vi "Main.vi"(7 "sweep rate, /min":dbl=0.2, 8 "sweep to:":dbl=-0.5, 9 "sweep":T6(radio)=enum."time_sweep") -> ()   [LabVIEW 2017] (continued)
                    n2924 = Build Array(w3784) -> (w3785:string[])
                    n2925 = property on="data_caption" class="Str"("Value"=w3787) -> ()  [unwired: 2 in, 2 out]
                    n2926 = property on="Figure_axis" class="Arr (strict)"("Value"=w3785) -> ()  [unwired: 2 in, 2 out]
                  }
                }
              }
              frame "2636a_smub" {
                n2927 = stacked-sequence {
                  frame #0 {
                    n2928 = property on="data_caption" class="Str"("Value"="") -> ()  [unwired: 2 in, 2 out]
                    n2929 = property on="Figure_axis" class="Arr (strict)"("Value"=string[] [] ("Figure_axis_string")) -> ()  [unwired: 2 in, 2 out]
                  }
                  frame #1 {
                    w3790 = "V_sweep_2636a_smub" ("V_sweep")
                    n2930 = Build Array(w3790) -> (w3791:string[])
                    n2931 = Concatenate Strings(w3790, "\t") -> (w3793:string)
                    n2932 = property on="Figure_axis" class="Arr (strict)"("Value"=w3791) -> ()  [unwired: 2 in, 2 out]
                    n2933 = property on="data_caption" class="Str"("Value"=w3793) -> ()  [unwired: 2 in, 2 out]
                  }
                }
              }
              frame "time_sweep", Default {
                n2934 = stacked-sequence {
                  frame #0 {
                    n2935 = property on="data_caption" class="Str"("Value"="") -> ()  [unwired: 2 in, 2 out]
                    n2936 = property on="Figure_axis" class="Arr (strict)"("Value"=string[] [] ("Figure_axis_string")) -> ()  [unwired: 2 in, 2 out]
                  }
                  frame #1 {
                    w3796 = "time_sweep" ("V_sweep")
                    n2937 = Build Array(w3796) -> (w3797:string[])
                    n2938 = Concatenate Strings(w3796, "\t") -> (w3798:string)
                    n2939 = property on="Figure_axis" class="Arr (strict)"("Value"=w3797) -> ()  [unwired: 2 in, 2 out]
                    n2940 = property on="data_caption" class="Str"("Value"=w3798) -> ()  [unwired: 2 in, 2 out]
                  }
                }
              }
              frame "iPS" {
                n2941 = stacked-sequence {
                  frame #0 {
                    n2942 = property on="data_caption" class="Str"("Value"="") -> ()  [unwired: 2 in, 2 out]
                    n2943 = property on="Figure_axis" class="Arr (strict)"("Value"=string[] [] ("Figure_axis_string")) -> ()  [unwired: 2 in, 2 out]
                  }
                  frame #1 {
                    w3802 = "Teslatron_iPS_OutputField" ("V_sweep")
                    n2944 = Build Array(w3802) -> (w3803:string[])
                    n2945 = Concatenate Strings(w3802, "\t") -> (w3805:string)
                    n2946 = property on="Figure_axis" class="Arr (strict)"("Value"=w3803) -> ()  [unwired: 2 in, 2 out]
                    n2947 = property on="data_caption" class="Str"("Value"=w3805) -> ()  [unwired: 2 in, 2 out]
                  }
                }
              }
              frame "iTC" {
                n2948 = stacked-sequence {
                  frame #0 {
                    n2949 = property on="data_caption" class="Str"("Value"="") -> ()  [unwired: 2 in, 2 out]
                    n2950 = property on="Figure_axis" class="Arr (strict)"("Value"=string[] ["", "SR830_1_ip", "SR830_1_oop", "SR830_2_ip", "SR830_2_oop", "2461_meas_v", "2461_meas_i", "2636A_smua_v", "2636A_smua_i", "formula"] ("Figure_axis")) -> ()  [unwired: 2 in, 2 out]
                  }
                  frame #1 {
                    w3810 = "Teslatron_iTC_Temp"
                    n2951 = Build Array(w3810) -> (w3809:string[])
                    n2952 = Concatenate Strings(w3810, "\t") -> (w3808:string)
                    n2953 = property on="data_caption" class="Str"("Value"=w3808) -> ()  [unwired: 2 in, 2 out]
                    n2954 = property on="Figure_axis" class="Arr (strict)"("Value"=w3809) -> ()  [unwired: 2 in, 2 out]
                  }
                }
              }
              frame "2461" {
                n2955 = stacked-sequence {
                  frame #0 {
                    n2956 = property on="data_caption" class="Str"("Value"="") -> ()  [unwired: 2 in, 2 out]
                    n2957 = property on="Figure_axis" class="Arr (strict)"("Value"=string[] ["", "SR830_1_ip", "SR830_1_oop", "SR830_2_ip", "SR830_2_oop", "2461_meas_v", "2461_meas_i", "2636A_smua_v", "2636A_smua_i", "formula"] ("Figure_axis")) -> ()  [unwired: 2 in, 2 out]
                  }
                  frame #1 {
                    w3816 = "I_sweep_2461"
                    n2958 = Build Array(w3816) -> (w3815:string[])
                    n2959 = Concatenate Strings(w3816, "\t") -> (w3814:string)
                    n2960 = property on="data_caption" class="Str"("Value"=w3814) -> ()  [unwired: 2 in, 2 out]
                    n2961 = property on="Figure_axis" class="Arr (strict)"("Value"=w3815) -> ()  [unwired: 2 in, 2 out]
                  }
                }
              }
            }
            n2962 = case shown="True" w3759 {
              frame False {
              }
              frame True {
                # "opens session for 2636a system sourcemeter"
                n2963 = local read "2336A addr"() -> (w3818:refnum<visa-resource-name>)
                n2964 = VISA Open(VISA resource name=w3818) -> ()  [unwired: 4 in, 2 out]
              }
            }
          }
          frame #1 {
            # "this part constructs the first (text) line for the data file with names of all measured variables,\nalso constructs a text array contaning names of all measured variable for the \"ring\" (so parameter can be selected and plotted)"
            n2965 = stacked-sequence {
              tunnel: [w3819 _ _ _ _ _ _ _ _ _ _ _ _ _ _ _ _ _ _ _ _ _ _ _ _ _ _ _ _ _ _ _ _ _ _ _ _ _ _ _ _ _ _ _ _ _ _ _ _ _ _ _] -> _
              frame #0 {
                # "SR830 1 in phase (SR830_1_ip)"
                n2966 = local read "SR830 1 ip"() -> (w3824:bool)
                n2967 = property on="Figure_axis" class="Arr (strict)"() -> ("Value"=w3821:string[])  [unwired: 2 in, 2 out]
                n2968 = property on="data_caption" class="Str"() -> ("Value"=w3823:string)  [unwired: 2 in, 2 out]
                n2969 = case shown="True" w3824 {
                  tunnel: w3823 -> [w3826 w3832]
                  tunnel: [w3826 w3831] -> w3822
                  tunnel: w3821 -> [w3825 w3829]
                  tunnel: [w3825 w3827] -> w3820
                  frame False {
                    # "not measure SR830 1 in phase signal (SR830_1_ip)"
                  }
                  frame True {
                    w3828 = "SR830_1_ip"
                    # "measure SR830 1 in phase signal (SR830_1_ip)"
                    n2970 = local read "SR830 1 addr"() -> (w3833:u8)
                    n2971 = Number To Decimal String(number=w3833) -> (decimal integer string=w3834:string)  [unwired: 1 in]
                    n2972 = GPIB Clear(3:w3834) -> ()  [unwired: 1 in, 2 out]
                    n2973 = Build Array (concatenate)(w3829, w3828) -> (w3827:string[])
                    n2974 = Concatenate Strings(w3832, w3828, "\t") -> (w3831:string)
                  }
                }
                n2975 = property on="Figure_axis" class="Arr (strict)"("Value"=w3820) -> ()  [unwired: 2 in, 2 out]
                n2976 = property on="data_caption" class="Str"("Value"=w3822) -> (error out=w3819:errorcluster)  [unwired: 2 in, 1 out]
              }
              frame #1 {
                # "SR830 1 out of phase (SR830_1_oop)"
                n2977 = local read "SR830 1 oop"() -> (w3839:bool)
                n2978 = property on="Figure_axis" class="Arr (strict)"() -> ("Value"=w3836:string[])  [unwired: 2 in, 2 out]
                n2979 = property on="data_caption" class="Str"() -> ("Value"=w3838:string)  [unwired: 2 in, 2 out]
                n2980 = case shown="False" w3839 {
                  tunnel: w3838 -> [w3841 w3847]
                  tunnel: [w3841 w3846] -> w3837
                  tunnel: w3836 -> [w3840 w3844]
                  tunnel: [w3840 w3842] -> w3835
                  frame False {
                    # "not measure SR830 1 out of phase signal (SR830_1_oop)"
                  }
                  frame True {
                    w3843 = "SR830_1_oop"
                    # "measure SR830 1 out of phase signal (SR830_1_oop)"
                    n2981 = local read "SR830 1 addr"() -> (w3848:u8)
                    n2982 = Number To Decimal String(number=w3848) -> (decimal integer string=w3849:string)  [unwired: 1 in]
                    n2983 = GPIB Clear(3:w3849) -> ()  [unwired: 1 in, 2 out]
                    n2984 = Build Array (concatenate)(w3844, w3843) -> (w3842:string[])
                    n2985 = Concatenate Strings(w3847, w3843, "\t") -> (w3846:string)
                  }
                }
                n2986 = property on="Figure_axis" class="Arr (strict)"("Value"=w3835) -> ()  [unwired: 2 in, 2 out]
                n2987 = property on="data_caption" class="Str"("Value"=w3837) -> ()  [unwired: 2 in, 2 out]
              }
              frame #2 {
                # "SR830 2 in phase (SR830_2_ip)"
                n2988 = local read "SR830 2 ip"() -> (w3854:bool)
                n2989 = property on="Figure_axis" class="Arr (strict)"() -> ("Value"=w3851:string[])  [unwired: 2 in, 2 out]
                n2990 = property on="data_caption" class="Str"() -> ("Value"=w3853:string)  [unwired: 2 in, 2 out]
                n2991 = case shown="True" w3854 {
                  tunnel: w3853 -> [w3856 w3862]
                  tunnel: [w3856 w3861] -> w3852
                  tunnel: w3851 -> [w3855 w3859]
                  tunnel: [w3855 w3857] -> w3850
                  frame False {
                    # "not measure SR830 2 in phase signal (SR830_2_ip)"
                  }
                  frame True {
                    w3858 = "SR830_2_ip"
                    # "measure SR830 2 in phase signal (SR830_2_ip)"
                    n2992 = local read "SR830 2 addr"() -> (w3863:u8)
                    n2993 = Number To Decimal String(number=w3863) -> (decimal integer string=w3864:string)  [unwired: 1 in]
                    n2994 = GPIB Clear(3:w3864) -> ()  [unwired: 1 in, 2 out]
                    n2995 = Build Array (concatenate)(w3859, w3858) -> (w3857:string[])
                    n2996 = Concatenate Strings(w3862, w3858, "\t") -> (w3861:string)
                  }
                }
                n2997 = property on="Figure_axis" class="Arr (strict)"("Value"=w3850) -> ()  [unwired: 2 in, 2 out]
                n2998 = property on="data_caption" class="Str"("Value"=w3852) -> ()  [unwired: 2 in, 2 out]
              }
              frame #3 {
                # "SR830 2 out of phase (SR830_2_oop)"
                n2999 = local read "SR830 2 oop"() -> (w3869:bool)
                n3000 = property on="Figure_axis" class="Arr (strict)"() -> ("Value"=w3866:string[])  [unwired: 2 in, 2 out]
                n3001 = property on="data_caption" class="Str"() -> ("Value"=w3868:string)  [unwired: 2 in, 2 out]
                n3002 = case shown="False" w3869 {
                  tunnel: w3868 -> [w3871 w3877]
                  tunnel: [w3871 w3876] -> w3867
                  tunnel: w3866 -> [w3870 w3874]
                  tunnel: [w3870 w3872] -> w3865
                  frame False {
                    # "not measure SR830 2 out of phase signal (SR830_2_oop)"
                  }
                  frame True {
                    w3873 = "SR830_2_oop"
                    # "measure SR830 2 out of phase signal (SR830_2_oop)"
                    n3003 = local read "SR830 2 addr"() -> (w3878:u8)
                    n3004 = Number To Decimal String(number=w3878) -> (decimal integer string=w3879:string)  [unwired: 1 in]
                    n3005 = GPIB Clear(3:w3879) -> ()  [unwired: 1 in, 2 out]
                    n3006 = Build Array (concatenate)(w3874, w3873) -> (w3872:string[])
                    n3007 = Concatenate Strings(w3877, w3873, "\t") -> (w3876:string)
                  }
                }
                n3008 = property on="Figure_axis" class="Arr (strict)"("Value"=w3865) -> ()  [unwired: 2 in, 2 out]
                n3009 = property on="data_caption" class="Str"("Value"=w3867) -> ()  [unwired: 2 in, 2 out]
              }
              frame #4 {
                # "SR830 3 in phase (SR830_3_ip)"
                n3010 = local read "SR830 3 ip"() -> (w3884:bool)
                n3011 = property on="Figure_axis" class="Arr (strict)"() -> ("Value"=w3881:string[])  [unwired: 2 in, 2 out]
                n3012 = property on="data_caption" class="Str"() -> ("Value"=w3883:string)  [unwired: 2 in, 2 out]
                n3013 = case shown="True" w3884 {
                  tunnel: w3883 -> [w3886 w3892]
                  tunnel: [w3886 w3891] -> w3882
                  tunnel: w3881 -> [w3885 w3889]
                  tunnel: [w3885 w3887] -> w3880
                  frame False {
                    # "not measure SR830 3 in phase signal (SR830_3_ip)"
                  }
                  frame True {
                    w3888 = "SR830_3_ip"
                    # "measure SR830 3 in phase signal (SR830_3_ip)"
                    n3014 = local read "SR830 3 addr"() -> (w3893:u8)
                    n3015 = Number To Decimal String(number=w3893) -> (decimal integer string=w3894:string)  [unwired: 1 in]
                    n3016 = GPIB Clear(3:w3894) -> ()  [unwired: 1 in, 2 out]
                    n3017 = Build Array (concatenate)(w3889, w3888) -> (w3887:string[])
                    n3018 = Concatenate Strings(w3892, w3888, "\t") -> (w3891:string)
                  }
                }
                n3019 = property on="Figure_axis" class="Arr (strict)"("Value"=w3880) -> ()  [unwired: 2 in, 2 out]
                n3020 = property on="data_caption" class="Str"("Value"=w3882) -> ()  [unwired: 2 in, 2 out]
              }
              frame #5 {
                # "SR830 3 out of phase (SR830_3_oop)"
                n3021 = local read "SR830 3 oop"() -> (w3899:bool)
                n3022 = property on="Figure_axis" class="Arr (strict)"() -> ("Value"=w3896:string[])  [unwired: 2 in, 2 out]
                n3023 = property on="data_caption" class="Str"() -> ("Value"=w3898:string)  [unwired: 2 in, 2 out]
                n3024 = case shown="True" w3899 {
                  tunnel: w3898 -> [w3901 w3907]
                  tunnel: [w3901 w3906] -> w3897
                  tunnel: w3896 -> [w3900 w3904]
                  tunnel: [w3900 w3902] -> w3895
                  frame False {
                    # "not measure SR830 3 out of phase signal (SR830_3_oop)"
                  }
                  frame True {
                    w3903 = "SR830_3_oop"
                    # "measure SR830 3 out phase signal (SR830_3_oop)"
                    n3025 = local read "SR830 3 addr"() -> (w3908:u8)
                    n3026 = Number To Decimal String(number=w3908) -> (decimal integer string=w3909:string)  [unwired: 1 in]
                    n3027 = GPIB Clear(3:w3909) -> ()  [unwired: 1 in, 2 out]
                    n3028 = Build Array (concatenate)(w3904, w3903) -> (w3902:string[])
                    n3029 = Concatenate Strings(w3907, w3903, "\t") -> (w3906:string)
                  }
                }
                n3030 = property on="Figure_axis" class="Arr (strict)"("Value"=w3895) -> ()  [unwired: 2 in, 2 out]
                n3031 = property on="data_caption" class="Str"("Value"=w3897) -> ()  [unwired: 2 in, 2 out]
              }
              frame #6 {
                # "SR830 4 in phase (SR830_4_ip)"
                n3032 = local read "SR830 4 ip"() -> (w3914:bool)
                n3033 = property on="Figure_axis" class="Arr (strict)"() -> ("Value"=w3911:string[])  [unwired: 2 in, 2 out]
                n3034 = property on="data_caption" class="Str"() -> ("Value"=w3913:string)  [unwired: 2 in, 2 out]
                n3035 = case shown="False" w3914 {
                  tunnel: w3913 -> [w3916 w3922]
                  tunnel: [w3916 w3921] -> w3912
                  tunnel: w3911 -> [w3915 w3919]
                  tunnel: [w3915 w3917] -> w3910
                  frame False {
                    # "not measure SR830 4 in phase signal (SR830_4_ip)"
                  }
                  frame True {
                    w3918 = "SR830_4_ip"
                    # "measure SR830 4 in phase signal (SR830_4_ip)"
                    n3036 = local read "SR830 4 addr"() -> (w3923:u8)
                    n3037 = Number To Decimal String(number=w3923) -> (decimal integer string=w3924:string)  [unwired: 1 in]
                    n3038 = GPIB Clear(3:w3924) -> ()  [unwired: 1 in, 2 out]
                    n3039 = Build Array (concatenate)(w3919, w3918) -> (w3917:string[])
                    n3040 = Concatenate Strings(w3922, w3918, "\t") -> (w3921:string)
                  }
                }
                n3041 = property on="Figure_axis" class="Arr (strict)"("Value"=w3910) -> ()  [unwired: 2 in, 2 out]
                n3042 = property on="data_caption" class="Str"("Value"=w3912) -> ()  [unwired: 2 in, 2 out]
              }
              frame #7 {
                # "SR830 4 out of phase (SR830_4_oop)"
                n3043 = local read "SR830 4 oop"() -> (w3929:bool)
                n3044 = property on="Figure_axis" class="Arr (strict)"() -> ("Value"=w3926:string[])  [unwired: 2 in, 2 out]
                n3045 = property on="data_caption" class="Str"() -> ("Value"=w3928:string)  [unwired: 2 in, 2 out]
                n3046 = case shown="False" w3929 {
                  tunnel: w3928 -> [w3931 w3937]
                  tunnel: [w3931 w3936] -> w3927
                  tunnel: w3926 -> [w3930 w3934]
                  tunnel: [w3930 w3932] -> w3925
                  frame False {
                    # "not measure SR830 4 out of phase signal (SR830_4_oop)"
                  }
                  frame True {
                    w3933 = "SR830_4_oop"
                    # "measure SR830 4 out of phase signal (SR830_4_oop)"
                    n3047 = local read "SR830 4 addr"() -> (w3938:u8)
                    n3048 = Number To Decimal String(number=w3938) -> (decimal integer string=w3939:string)  [unwired: 1 in]
                    n3049 = GPIB Clear(3:w3939) -> ()  [unwired: 1 in, 2 out]
                    n3050 = Build Array (concatenate)(w3934, w3933) -> (w3932:string[])
                    n3051 = Concatenate Strings(w3937, w3933, "\t") -> (w3936:string)
                  }
                }
                n3052 = property on="Figure_axis" class="Arr (strict)"("Value"=w3925) -> ()  [unwired: 2 in, 2 out]
                n3053 = property on="data_caption" class="Str"("Value"=w3927) -> ()  [unwired: 2 in, 2 out]
              }
              frame #8 {
                # "SR830 5 in phase (SR830_5_ip)"
                n3054 = local read "SR830 5 ip"() -> (w3944:bool)
                n3055 = property on="Figure_axis" class="Arr (strict)"() -> ("Value"=w3941:string[])  [unwired: 2 in, 2 out]
                n3056 = property on="data_caption" class="Str"() -> ("Value"=w3943:string)  [unwired: 2 in, 2 out]
                n3057 = case shown="True" w3944 {
                  tunnel: w3943 -> [w3946 w3952]
                  tunnel: [w3946 w3951] -> w3942
                  tunnel: w3941 -> [w3945 w3949]
                  tunnel: [w3945 w3947] -> w3940
                  frame False {
                    # "not measure SR830 5 in phase signal (SR830_5_ip)"
                  }
                  frame True {
                    w3948 = "SR830_5_ip"
                    # "measure SR830 5 in phase signal (SR830_5_ip)"
                    n3058 = local read "SR830 5 addr"() -> (w3953:u8)
                    n3059 = Number To Decimal String(number=w3953) -> (decimal integer string=w3954:string)  [unwired: 1 in]
                    n3060 = GPIB Clear(3:w3954) -> ()  [unwired: 1 in, 2 out]
                    n3061 = Build Array (concatenate)(w3949, w3948) -> (w3947:string[])
                    n3062 = Concatenate Strings(w3952, w3948, "\t") -> (w3951:string)
                  }
                }
                n3063 = property on="Figure_axis" class="Arr (strict)"("Value"=w3940) -> ()  [unwired: 2 in, 2 out]
                n3064 = property on="data_caption" class="Str"("Value"=w3942) -> ()  [unwired: 2 in, 2 out]
              }
              frame #9 {
                # "SR830 5 out of phase (SR830_5_oop)"
                n3065 = local read "SR830 5 oop"() -> (w3959:bool)
                n3066 = property on="Figure_axis" class="Arr (strict)"() -> ("Value"=w3956:string[])  [unwired: 2 in, 2 out]
                n3067 = property on="data_caption" class="Str"() -> ("Value"=w3958:string)  [unwired: 2 in, 2 out]
                n3068 = case shown="True" w3959 {
                  tunnel: w3958 -> [w3961 w3967]
                  tunnel: [w3961 w3966] -> w3957
                  tunnel: w3956 -> [w3960 w3964]
                  tunnel: [w3960 w3962] -> w3955
                  frame False {
                    # "not measure SR830 5 out of phase signal (SR830_5_oop)"
                  }
                  frame True {
                    w3963 = "SR830_5_oop"
                    # "measure SR830 5 out of phase signal (SR830_5_oop)"
                    n3069 = local read "SR830 5 addr"() -> (w3968:u8)
                    n3070 = Number To Decimal String(number=w3968) -> (decimal integer string=w3969:string)  [unwired: 1 in]
                    n3071 = GPIB Clear(3:w3969) -> ()  [unwired: 1 in, 2 out]
                    n3072 = Build Array (concatenate)(w3964, w3963) -> (w3962:string[])
                    n3073 = Concatenate Strings(w3967, w3963, "\t") -> (w3966:string)
                  }
                }
                n3074 = property on="Figure_axis" class="Arr (strict)"("Value"=w3955) -> ()  [unwired: 2 in, 2 out]
                n3075 = property on="data_caption" class="Str"("Value"=w3957) -> ()  [unwired: 2 in, 2 out]
              }
              frame #10 {
                # "SR830 6 in phase (SR830_6_ip)"
                n3076 = property on="SR830_6_ip" class="Bool (strict)"() -> ("Value"=w3970:bool)  [unwired: 2 in, 2 out]
                n3077 = property on="Figure_axis" class="Arr (strict)"() -> ("Value"=w3972:string[])  [unwired: 2 in, 2 out]
                n3078 = property on="data_caption" class="Str"() -> ("Value"=w3974:string)  [unwired: 2 in, 2 out]
                n3079 = case shown="True" w3970 {
                  tunnel: w3974 -> [w3976 w3982]
                  tunnel: [w3976 w3981] -> w3973
                  tunnel: w3972 -> [w3975 w3979]
                  tunnel: [w3975 w3977] -> w3971
                  frame False {
                    # "not measure SR830 6 in phase signal (SR830_6_ip)"
                  }
                  frame True {
                    w3978 = "SR830_6_ip"
                    # "measure SR830 6 in phase signal (SR830_6_ip)"
                    n3080 = local read "SR830_6"() -> (w3983:u8)
                    n3081 = Number To Decimal String(number=w3983) -> (decimal integer string=w3984:string)  [unwired: 1 in]
                    n3082 = GPIB Clear(3:w3984) -> ()  [unwired: 1 in, 2 out]
                    n3083 = Build Array (concatenate)(w3979, w3978) -> (w3977:string[])
                    n3084 = Concatenate Strings(w3982, w3978, "\t") -> (w3981:string)
                  }
                }
                n3085 = property on="Figure_axis" class="Arr (strict)"("Value"=w3971) -> ()  [unwired: 2 in, 2 out]
                n3086 = property on="data_caption" class="Str"("Value"=w3973) -> ()  [unwired: 2 in, 2 out]
              }
              frame #11 {
                # "SR830 6 out of phase (SR830_6_oop)"
                n3087 = local read "SR830_6_oop"() -> (w3989:bool)
                n3088 = property on="Figure_axis" class="Arr (strict)"() -> ("Value"=w3986:string[])  [unwired: 2 in, 2 out]
                n3089 = property on="data_caption" class="Str"() -> ("Value"=w3988:string)  [unwired: 2 in, 2 out]
                n3090 = case shown="False" w3989 {
                  tunnel: w3988 -> [w3991 w3997]
                  tunnel: [w3991 w3996] -> w3987
                  tunnel: w3986 -> [w3990 w3994]
                  tunnel: [w3990 w3992] -> w3985
                  frame False {
                    # "not measure SR830 6 out of phase signal (SR830_6_oop)"
                  }
                  frame True {
                    w3993 = "SR830_6_oop"
                    # "measure SR830 6 out of phase signal (SR830_6_oop)"
                    n3091 = local read "SR830_6"() -> (w3998:u8)
                    n3092 = Number To Decimal String(number=w3998) -> (decimal integer string=w3999:string)  [unwired: 1 in]
                    n3093 = GPIB Clear(3:w3999) -> ()  [unwired: 1 in, 2 out]
                    n3094 = Build Array (concatenate)(w3994, w3993) -> (w3992:string[])
                    n3095 = Concatenate Strings(w3997, w3993, "\t") -> (w3996:string)
                  }
                }
                n3096 = property on="Figure_axis" class="Arr (strict)"("Value"=w3985) -> ()  [unwired: 2 in, 2 out]
                n3097 = property on="data_caption" class="Str"("Value"=w3987) -> ()  [unwired: 2 in, 2 out]
              }
              frame #12 {
                # "SR830 7 in phase (SR830_7_ip)"
                n3098 = local read "SR830_7_ip"() -> (w4000:bool)
                n3099 = property on="Figure_axis" class="Arr (strict)"() -> ("Value"=w4002:string[])  [unwired: 2 in, 2 out]
                n3100 = property on="data_caption" class="Str"() -> ("Value"=w4004:string)  [unwired: 2 in, 2 out]
                n3101 = case shown="True" w4000 {
                  tunnel: w4004 -> [w4006 w4012]
                  tunnel: [w4006 w4011] -> w4003
                  tunnel: w4002 -> [w4005 w4009]
                  tunnel: [w4005 w4007] -> w4001
                  frame False {
                    # "not measure SR830 7 in phase signal (SR830_7_ip)"
                  }
                  frame True {
                    w4008 = "SR830_7_ip"
                    # "measure SR830 7 in phase signal (SR830_7_ip)"
                    n3102 = local read "SR830_7"() -> (w4013:u8)
                    n3103 = Number To Decimal String(number=w4013) -> (decimal integer string=w4014:string)  [unwired: 1 in]
                    n3104 = GPIB Clear(3:w4014) -> ()  [unwired: 1 in, 2 out]
                    n3105 = Build Array (concatenate)(w4009, w4008) -> (w4007:string[])
                    n3106 = Concatenate Strings(w4012, w4008, "\t") -> (w4011:string)
                  }
                }
                n3107 = property on="Figure_axis" class="Arr (strict)"("Value"=w4001) -> ()  [unwired: 2 in, 2 out]
                n3108 = property on="data_caption" class="Str"("Value"=w4003) -> ()  [unwired: 2 in, 2 out]
              }
              frame #13 {
                # "SR830 7 out of phase (SR830_7_oop)"
                n3109 = local read "SR830_7_oop"() -> (w4019:bool)
                n3110 = property on="Figure_axis" class="Arr (strict)"() -> ("Value"=w4016:string[])  [unwired: 2 in, 2 out]
                n3111 = property on="data_caption" class="Str"() -> ("Value"=w4018:string)  [unwired: 2 in, 2 out]
                n3112 = case shown="True" w4019 {
                  tunnel: w4018 -> [w4021 w4027]
                  tunnel: [w4021 w4026] -> w4017
                  tunnel: w4016 -> [w4020 w4024]
                  tunnel: [w4020 w4022] -> w4015
                  frame False {
                    # "not measure SR830 7 out of phase signal (SR830_7_oop)"
                  }
                  frame True {
                    w4023 = "SR830_7_oop"
                    # "measure SR830 7 out of phase signal (SR830_7_oop)"
                    n3113 = local read "SR830_7"() -> (w4028:u8)
                    n3114 = Number To Decimal String(number=w4028) -> (decimal integer string=w4029:string)  [unwired: 1 in]
                    n3115 = GPIB Clear(3:w4029) -> ()  [unwired: 1 in, 2 out]
                    n3116 = Build Array (concatenate)(w4024, w4023) -> (w4022:string[])
                    n3117 = Concatenate Strings(w4027, w4023, "\t") -> (w4026:string)
                  }
                }
                n3118 = property on="Figure_axis" class="Arr (strict)"("Value"=w4015) -> ()  [unwired: 2 in, 2 out]
                n3119 = property on="data_caption" class="Str"("Value"=w4017) -> ()  [unwired: 2 in, 2 out]
              }
              frame #14 {
                # "SR830 8 in phase (SR830_8_ip)"
                n3120 = local read "SR830_8_ip"() -> (w4030:bool)
                n3121 = property on="Figure_axis" class="Arr (strict)"() -> ("Value"=w4032:string[])  [unwired: 2 in, 2 out]
                n3122 = property on="data_caption" class="Str"() -> ("Value"=w4034:string)  [unwired: 2 in, 2 out]
                n3123 = case shown="True" w4030 {
                  tunnel: w4034 -> [w4036 w4042]
                  tunnel: [w4036 w4041] -> w4033
                  tunnel: w4032 -> [w4035 w4039]
                  tunnel: [w4035 w4037] -> w4031
                  frame False {
                    # "not measure SR830 8 in phase signal (SR830_8_ip)"
                  }
                  frame True {
                    w4038 = "SR830_8_ip"
                    # "measure SR830 8 in phase signal (SR830_8_ip)"
                    n3124 = local read "SR830_8"() -> (w4043:u8)
                    n3125 = Number To Decimal String(number=w4043) -> (decimal integer string=w4044:string)  [unwired: 1 in]
                    n3126 = GPIB Clear(3:w4044) -> ()  [unwired: 1 in, 2 out]
                    n3127 = Build Array (concatenate)(w4039, w4038) -> (w4037:string[])
                    n3128 = Concatenate Strings(w4042, w4038, "\t") -> (w4041:string)
                  }
                }
                n3129 = property on="Figure_axis" class="Arr (strict)"("Value"=w4031) -> ()  [unwired: 2 in, 2 out]
                n3130 = property on="data_caption" class="Str"("Value"=w4033) -> ()  [unwired: 2 in, 2 out]
              }
              frame #15 {
                # "SR830 8 out phase (SR830_8_oop)"
                n3131 = local read "SR830_8_oop"() -> (w4045:bool)
                n3132 = property on="Figure_axis" class="Arr (strict)"() -> ("Value"=w4047:string[])  [unwired: 2 in, 2 out]
                n3133 = property on="data_caption" class="Str"() -> ("Value"=w4049:string)  [unwired: 2 in, 2 out]
                n3134 = case shown="True" w4045 {
                  tunnel: w4049 -> [w4051 w4057]
                  tunnel: [w4051 w4056] -> w4048
                  tunnel: w4047 -> [w4050 w4054]
                  tunnel: [w4050 w4052] -> w4046
                  frame False {
                    # "not measure SR830 8 out phase signal (SR830_8_oop)"
                  }
                  frame True {
                    w4053 = "SR830_8_oop"
                    # "measure SR830 8 out phase signal (SR830_8_00p)"
                    n3135 = local read "SR830_8"() -> (w4058:u8)
                    n3136 = Number To Decimal String(number=w4058) -> (decimal integer string=w4059:string)  [unwired: 1 in]
                    n3137 = GPIB Clear(3:w4059) -> ()  [unwired: 1 in, 2 out]
                    n3138 = Build Array (concatenate)(w4054, w4053) -> (w4052:string[])
                    n3139 = Concatenate Strings(w4057, w4053, "\t") -> (w4056:string)
                  }
                }
                n3140 = property on="Figure_axis" class="Arr (strict)"("Value"=w4046) -> ()  [unwired: 2 in, 2 out]
                n3141 = property on="data_caption" class="Str"("Value"=w4048) -> ()  [unwired: 2 in, 2 out]
              }
              frame #16 {
                # "MFLI_V1"
                n3142 = property on="MFLI_1" class="Str" props=["Value"]() -> ()  [unwired: 2 in, 3 out]
                n3143 = property on="MFLI_V1" class="Bool (strict)"() -> ("Value"=w4060:bool)  [unwired: 2 in, 2 out]
                n3144 = property on="data_caption" class="Str"() -> ("Value"=w4064:string)  [unwired: 2 in, 2 out]
                n3145 = property on="Figure_axis" class="Arr (strict)"() -> ("Value"=w4062:string[])  [unwired: 2 in, 2 out]
                n3146 = case shown="True" w4060 {
                  tunnel: w4064 -> [w4066 w4076]
                  tunnel: [w4066 w4075] -> w4063
                  tunnel: w4062 -> [w4065 w4074]
                  tunnel: [w4065 w4073] -> w4061
                  frame False {
                    # "not measure 2461 voltage (2461_meas_v)"
                  }
                  frame True {
                    w4071 = "MFLI_Vy_1"
                    w4072 = "MFLI_Vx_1"
                    w4070 = "\t"
                    w4069 = "MFLI_freq_1"
                    n3147 = property on="HandleOut" class="Clust (strict)"() -> ("Value"=w4068:T5)  [unwired: 2 in, 2 out]
                    n3148 = Unbundle(w4068) -> ("Connected"=w4067:bool)  [unwired: 5 out]
                    n3149 = case shown="False" w4067 {
                      frame False {
                        n3150 = property on="MFLI_1" class="Str"() -> ("Value"=w4079:string)  [unwired: 2 in, 2 out]
                        n3151 = call <instrlib>:"ziOpen.vi"("Address"=w4079) -> ("HandleOut"=w4078:T5)  [unwired: 3 in, 2 out]
                        n3152 = call <instrlib>:"ziCheckVersion.vi"("Handle In"=w4078) -> ("Handle Out"=w4077:T5)  [unwired: 12 in, 2 out]
                        n3153 = property on="HandleOut" class="Clust (strict)"("Value"=w4077) -> ()  [unwired: 2 in, 2 out]
                      }
                      frame True {
                      }
                    }
                    n3154 = Build Array (concatenate)(w4074, w4072, w4071, w4069) -> (w4073:string[])
                    n3155 = Concatenate Strings(w4076, w4072, w4070, w4071, w4070, w4069, w4070) -> (w4075:string)
                  }
                }
                n3156 = property on="Figure_axis" class="Arr (strict)"("Value"=w4061) -> ()  [unwired: 2 in, 2 out]
                n3157 = property on="data_caption" class="Str"("Value"=w4063) -> ()  [unwired: 2 in, 2 out]
              }
              frame #17 {
                # "MFLI_I1"
                n3158 = property on="MFLI_I1" class="Bool (strict)"() -> ("Value"=w4080:bool)  [unwired: 2 in, 2 out]
                n3159 = property on="data_caption" class="Str"() -> ("Value"=w4084:string)  [unwired: 2 in, 2 out]
                n3160 = property on="Figure_axis" class="Arr (strict)"() -> ("Value"=w4082:string[])  [unwired: 2 in, 2 out]
                n3161 = case shown="True" w4080 {
                  tunnel: w4084 -> [w4086 w4096]
                  tunnel: [w4086 w4095] -> w4083
                  tunnel: w4082 -> [w4085 w4094]
                  tunnel: [w4085 w4093] -> w4081
                  frame False {
                    # "not measure 2461 voltage (2461_meas_v)"
                  }
                  frame True {
                    w4091 = "MFLI_Iy-1"
                    w4092 = "MFLI_Ix_1"
                    w4090 = "\t"
                    w4089 = "MFLI_freq_1"
                    n3162 = property on="HandleOut" class="Clust (strict)"() -> ("Value"=w4088:T5)  [unwired: 2 in, 2 out]
                    n3163 = Unbundle(w4088) -> ("Connected"=w4087:bool)  [unwired: 5 out]
                    n3164 = case shown="False" w4087 {
                      frame False {
                        n3165 = property on="MFLI_1" class="Str"() -> ("Value"=w4099:string)  [unwired: 2 in, 2 out]
                        n3166 = call <instrlib>:"ziOpen.vi"("Address"=w4099) -> ("HandleOut"=w4098:T5)  [unwired: 3 in, 2 out]
                        n3167 = call <instrlib>:"ziCheckVersion.vi"("Handle In"=w4098) -> ("Handle Out"=w4097:T5)  [unwired: 12 in, 2 out]
                        n3168 = property on="HandleOut" class="Clust (strict)"("Value"=w4097) -> ()  [unwired: 2 in, 2 out]
                      }
                      frame True {
                      }
                    }
                    n3169 = Build Array (concatenate)(w4094, w4092, w4091, w4089) -> (w4093:string[])
                    n3170 = Concatenate Strings(w4096, w4092, w4090, w4091, w4090, w4089, w4090) -> (w4095:string)
                  }
                }
                n3171 = property on="Figure_axis" class="Arr (strict)"("Value"=w4081) -> ()  [unwired: 2 in, 2 out]
                n3172 = property on="data_caption" class="Str"("Value"=w4083) -> ()  [unwired: 2 in, 2 out]
              }
              frame #18 {
                # "MFLI_V 2"
                n3173 = local read "MFLI_V2"() -> (w4100:bool)
                n3174 = property on="data_caption" class="Str"() -> ("Value"=w4104:string)  [unwired: 2 in, 2 out]
                n3175 = property on="Figure_axis" class="Arr (strict)"() -> ("Value"=w4102:string[])  [unwired: 2 in, 2 out]
                n3176 = case shown="True" w4100 {
                  tunnel: w4104 -> [w4106 w4116]
                  tunnel: [w4106 w4115] -> w4103
                  tunnel: w4102 -> [w4105 w4114]
                  tunnel: [w4105 w4113] -> w4101
                  frame False {
                  }
                  frame True {
                    w4111 = "MFLI_Vy_2"
                    w4112 = "MFLI_Vx_2"
                    w4110 = "\t"
                    w4109 = "MFLI_freq_2"
                    n3177 = property on="Handle Out 2" class="Clust (strict)"() -> ("Value"=w4108:T5)  [unwired: 2 in, 2 out]
                    n3178 = Unbundle(w4108) -> ("Connected"=w4107:bool)  [unwired: 5 out]
                    n3179 = case shown="False" w4107 {
                      frame False {
                        n3180 = local read "MFLI_2"() -> (w4117:string)
                        n3181 = call <instrlib>:"ziOpen.vi"("Address"=w4117) -> ("HandleOut"=w4119:T5)  [unwired: 3 in, 2 out]
                        n3182 = call <instrlib>:"ziCheckVersion.vi"("Handle In"=w4119) -> ("Handle Out"=w4118:T5)  [unwired: 12 in, 2 out]
                        n3183 = property on="Handle Out 2" class="Clust (strict)"("Value"=w4118) -> ()  [unwired: 2 in, 2 out]
                      }
                      frame True {
                      }
                    }
                    n3184 = Build Array (concatenate)(w4114, w4112, w4111, w4109) -> (w4113:string[])
                    n3185 = Concatenate Strings(w4116, w4112, w4110, w4111, w4110, w4109, w4110) -> (w4115:string)
                  }
                }
                n3186 = property on="Figure_axis" class="Arr (strict)"("Value"=w4101) -> ()  [unwired: 2 in, 2 out]
                n3187 = property on="data_caption" class="Str"("Value"=w4103) -> ()  [unwired: 2 in, 2 out]
              }
              frame #19 {
                # "MFLI_I 2"
                n3188 = local read "MFLI_I2"() -> (w4120:bool)
                n3189 = property on="data_caption" class="Str"() -> ("Value"=w4124:string)  [unwired: 2 in, 2 out]
                n3190 = property on="Figure_axis" class="Arr (strict)"() -> ("Value"=w4122:string[])  [unwired: 2 in, 2 out]
                n3191 = case shown="True" w4120 {
                  tunnel: w4124 -> [w4126 w4136]
                  tunnel: [w4126 w4135] -> w4123
                  tunnel: w4122 -> [w4125 w4134]
                  tunnel: [w4125 w4133] -> w4121
                  frame False {
                    # "not measure 2461 voltage (2461_meas_v)"
                  }
                  frame True {
                    w4131 = "MFLI_Iy_2"
                    w4132 = "MFLI_Ix_2"
                    w4130 = "\t"
                    w4129 = "MFLI_freq_2"
                    n3192 = property on="Handle Out 2" class="Clust (strict)"() -> ("Value"=w4128:T5)  [unwired: 2 in, 2 out]
                    n3193 = Unbundle(w4128) -> ("Connected"=w4127:bool)  [unwired: 5 out]
                    n3194 = case shown="False" w4127 {
                      frame False {
                        n3195 = local read "MFLI_2"() -> (w4137:string)
                        n3196 = call <instrlib>:"ziOpen.vi"("Address"=w4137) -> ("HandleOut"=w4139:T5)  [unwired: 3 in, 2 out]
                        n3197 = call <instrlib>:"ziCheckVersion.vi"("Handle In"=w4139) -> ("Handle Out"=w4138:T5)  [unwired: 12 in, 2 out]
                        n3198 = property on="Handle Out 2" class="Clust (strict)"("Value"=w4138) -> ()  [unwired: 2 in, 2 out]
                      }
                      frame True {
                      }
                    }
                    n3199 = Build Array (concatenate)(w4134, w4132, w4131, w4129) -> (w4133:string[])
                    n3200 = Concatenate Strings(w4136, w4132, w4130, w4131, w4130, w4129, w4130) -> (w4135:string)
                  }
                }
                n3201 = property on="Figure_axis" class="Arr (strict)"("Value"=w4121) -> ()  [unwired: 2 in, 2 out]
                n3202 = property on="data_caption" class="Str"("Value"=w4123) -> ()  [unwired: 2 in, 2 out]
              }
              frame #20 {
                # "2400 1 voltage measure (2400_1_v)"
                n3203 = local read "2400 1 meas v"() -> (w4144:bool)
                n3204 = property on="Figure_axis" class="Arr (strict)"() -> ("Value"=w4141:string[])  [unwired: 2 in, 2 out]
                n3205 = property on="data_caption" class="Str"() -> ("Value"=w4143:string)  [unwired: 2 in, 2 out]
                n3206 = case shown="False" w4144 {
                  tunnel: w4143 -> [w4146 w4152]
                  tunnel: [w4146 w4151] -> w4142
                  tunnel: w4141 -> [w4145 w4149]
                  tunnel: [w4145 w4147] -> w4140
                  frame False {
                    # "not measure 2400 1 voltage (2400_1_v)"
                  }
                  frame True {
                    w4148 = "2400_1_v"
                    # "measure 2400 1 voltage (2400_1_v)"
                    n3207 = local read "2400 1 addr"() -> (w4153:u8)
                    n3208 = Number To Decimal String(number=w4153) -> (decimal integer string=w4154:string)  [unwired: 1 in]
                    n3209 = GPIB Clear(3:w4154) -> ()  [unwired: 1 in, 2 out]
                    n3210 = Build Array (concatenate)(w4149, w4148) -> (w4147:string[])
                    n3211 = Concatenate Strings(w4152, w4148, "\t") -> (w4151:string)
                  }
                }
                n3212 = property on="Figure_axis" class="Arr (strict)"("Value"=w4140) -> ()  [unwired: 2 in, 2 out]
                n3213 = property on="data_caption" class="Str"("Value"=w4142) -> ()  [unwired: 2 in, 2 out]
              }
              frame #21 {
                # "2400 1 current measure (2400_1_i)"
                n3214 = local read "2400 1 meas i"() -> (w4159:bool)
                n3215 = property on="Figure_axis" class="Arr (strict)"() -> ("Value"=w4156:string[])  [unwired: 2 in, 2 out]
                n3216 = property on="data_caption" class="Str"() -> ("Value"=w4158:string)  [unwired: 2 in, 2 out]
                n3217 = case shown="False" w4159 {
                  tunnel: w4158 -> [w4161 w4167]
                  tunnel: [w4161 w4166] -> w4157
                  tunnel: w4156 -> [w4160 w4164]
                  tunnel: [w4160 w4162] -> w4155
                  frame False {
                    # "not measure 2400 1 current (2400_1_i)"
                  }
                  frame True {
                    w4163 = "2400_1_i"
                    # "measure 2400 1 current (2400_1_i)"
                    n3218 = local read "2400 1 addr"() -> (w4168:u8)
                    n3219 = Number To Decimal String(number=w4168) -> (decimal integer string=w4169:string)  [unwired: 1 in]
                    n3220 = GPIB Clear(3:w4169) -> ()  [unwired: 1 in, 2 out]
                    n3221 = Build Array (concatenate)(w4164, w4163) -> (w4162:string[])
                    n3222 = Concatenate Strings(w4167, w4163, "\t") -> (w4166:string)
                  }
                }
                n3223 = property on="Figure_axis" class="Arr (strict)"("Value"=w4155) -> ()  [unwired: 2 in, 2 out]
                n3224 = property on="data_caption" class="Str"("Value"=w4157) -> ()  [unwired: 2 in, 2 out]
              }
              frame #22 {
                # "2400 2 voltage measure (2400_2_v)"
                n3225 = local read "2400 2 meas v"() -> (w4174:bool)
                n3226 = property on="Figure_axis" class="Arr (strict)"() -> ("Value"=w4171:string[])  [unwired: 2 in, 2 out]
                n3227 = property on="data_caption" class="Str"() -> ("Value"=w4173:string)  [unwired: 2 in, 2 out]
                n3228 = case shown="False" w4174 {
                  tunnel: w4173 -> [w4176 w4182]
                  tunnel: [w4176 w4181] -> w4172
                  tunnel: w4171 -> [w4175 w4179]
                  tunnel: [w4175 w4177] -> w4170
                  frame False {
                    # "not measure 2400 2 voltage (2400_2_v)"
                  }
                  frame True {
                    w4178 = "2400_2_v"
                    # "measure 2400 2 voltage (2400_2_v)"
                    n3229 = local read "2400 2 addr"() -> (w4183:u8)
                    n3230 = Number To Decimal String(number=w4183) -> (decimal integer string=w4184:string)  [unwired: 1 in]
                    n3231 = GPIB Clear(3:w4184) -> ()  [unwired: 1 in, 2 out]
                    n3232 = Build Array (concatenate)(w4179, w4178) -> (w4177:string[])
                    n3233 = Concatenate Strings(w4182, w4178, "\t") -> (w4181:string)
                  }
                }
                n3234 = property on="Figure_axis" class="Arr (strict)"("Value"=w4170) -> ()  [unwired: 2 in, 2 out]
                n3235 = property on="data_caption" class="Str"("Value"=w4172) -> ()  [unwired: 2 in, 2 out]
              }
              frame #23 {
                # "2400 2 current measure (2400_2_i)"
                n3236 = local read "2400 2 meas i"() -> (w4189:bool)
                n3237 = property on="Figure_axis" class="Arr (strict)"() -> ("Value"=w4186:string[])  [unwired: 2 in, 2 out]
                n3238 = property on="data_caption" class="Str"() -> ("Value"=w4188:string)  [unwired: 2 in, 2 out]
                n3239 = case shown="False" w4189 {
                  tunnel: w4188 -> [w4191 w4197]
                  tunnel: [w4191 w4196] -> w4187
                  tunnel: w4186 -> [w4190 w4194]
                  tunnel: [w4190 w4192] -> w4185
                  frame False {
                    # "not measure 2400 2 current (2400_2_i)"
                  }
                  frame True {
                    w4193 = "2400_2_i"
                    # "measure 2400 2 current (2400_2_i)"
                    n3240 = local read "2400 2 addr"() -> (w4198:u8)
                    n3241 = Number To Decimal String(number=w4198) -> (decimal integer string=w4199:string)  [unwired: 1 in]
                    n3242 = GPIB Clear(3:w4199) -> ()  [unwired: 1 in, 2 out]
                    n3243 = Build Array (concatenate)(w4194, w4193) -> (w4192:string[])
                    n3244 = Concatenate Strings(w4197, w4193, "\t") -> (w4196:string)
                  }
                }
                n3245 = property on="Figure_axis" class="Arr (strict)"("Value"=w4185) -> ()  [unwired: 2 in, 2 out]
                n3246 = property on="data_caption" class="Str"("Value"=w4187) -> ()  [unwired: 2 in, 2 out]
              }
              frame #24 {
                # "2400 3 voltage measure (2400_3_v)"
                n3247 = local read "2400 3 meas v"() -> (w4204:bool)
                n3248 = property on="Figure_axis" class="Arr (strict)"() -> ("Value"=w4201:string[])  [unwired: 2 in, 2 out]
                n3249 = property on="data_caption" class="Str"() -> ("Value"=w4203:string)  [unwired: 2 in, 2 out]
                n3250 = case shown="False" w4204 {
                  tunnel: w4203 -> [w4206 w4212]
                  tunnel: [w4206 w4211] -> w4202
                  tunnel: w4201 -> [w4205 w4209]
                  tunnel: [w4205 w4207] -> w4200
                  frame False {
                    # "not measure 2400 3 voltage (2400_3_v)"
                  }
                  frame True {
                    w4208 = "2400_3_v"
                    # "measure 2400 3 voltage (2400_3_v)"
                    n3251 = local read "2400 3 addr"() -> (w4213:u8)
                    n3252 = Number To Decimal String(number=w4213) -> (decimal integer string=w4214:string)  [unwired: 1 in]
                    n3253 = GPIB Clear(3:w4214) -> ()  [unwired: 1 in, 2 out]
                    n3254 = Build Array (concatenate)(w4209, w4208) -> (w4207:string[])
                    n3255 = Concatenate Strings(w4212, w4208, "\t") -> (w4211:string)
                  }
                }
                n3256 = property on="Figure_axis" class="Arr (strict)"("Value"=w4200) -> ()  [unwired: 2 in, 2 out]
                n3257 = property on="data_caption" class="Str"("Value"=w4202) -> ()  [unwired: 2 in, 2 out]
              }
              frame #25 {
                # "2400 3 current measure (2400_3_i)"
                n3258 = local read "2400 3 meas i"() -> (w4219:bool)
                n3259 = property on="Figure_axis" class="Arr (strict)"() -> ("Value"=w4216:string[])  [unwired: 2 in, 2 out]
                n3260 = property on="data_caption" class="Str"() -> ("Value"=w4218:string)  [unwired: 2 in, 2 out]
                n3261 = case shown="True" w4219 {
                  tunnel: w4218 -> [w4221 w4227]
                  tunnel: [w4221 w4226] -> w4217
                  tunnel: w4216 -> [w4220 w4224]
                  tunnel: [w4220 w4222] -> w4215
                  frame False {
                    # "not measure 2400 3 current (2400_3_i)"
                  }
                  frame True {
                    w4223 = "2400_3_i"
                    # "measure 2400 3 current (2400_3_i)"
                    n3262 = local read "2400 3 addr"() -> (w4228:u8)
                    n3263 = Number To Decimal String(number=w4228) -> (decimal integer string=w4229:string)  [unwired: 1 in]
                    n3264 = GPIB Clear(3:w4229) -> ()  [unwired: 1 in, 2 out]
                    n3265 = Build Array (concatenate)(w4224, w4223) -> (w4222:string[])
                    n3266 = Concatenate Strings(w4227, w4223, "\t") -> (w4226:string)
                  }
                }
                n3267 = property on="Figure_axis" class="Arr (strict)"("Value"=w4215) -> ()  [unwired: 2 in, 2 out]
                n3268 = property on="data_caption" class="Str"("Value"=w4217) -> ()  [unwired: 2 in, 2 out]
              }
              frame #26 {
                # "2182A 1 channel 1 measure (2182A_1_ch1)"
                n3269 = local read "2182A 1 ch1"() -> (w4234:bool)
                n3270 = property on="Figure_axis" class="Arr (strict)"() -> ("Value"=w4231:string[])  [unwired: 2 in, 2 out]
                n3271 = property on="data_caption" class="Str"() -> ("Value"=w4233:string)  [unwired: 2 in, 2 out]
                n3272 = case shown="False" w4234 {
                  tunnel: w4233 -> [w4236 w4242]
                  tunnel: [w4236 w4241] -> w4232
                  tunnel: w4231 -> [w4235 w4239]
                  tunnel: [w4235 w4237] -> w4230
                  frame False {
                    # "not measure 2182A 1 channel 1 (2182A_1_ch1)"
                  }
                  frame True {
                    w4238 = "2182A_1_ch1"
                    # "measure 2182A 1 channel 1 (2182A_1_ch1)"
                    n3273 = local read "2182A 1 addr"() -> (w4243:u8)
                    n3274 = Number To Decimal String(number=w4243) -> (decimal integer string=w4244:string)  [unwired: 1 in]
                    n3275 = GPIB Clear(3:w4244) -> ()  [unwired: 1 in, 2 out]
                    n3276 = Build Array (concatenate)(w4239, w4238) -> (w4237:string[])
                    n3277 = Concatenate Strings(w4242, w4238, "\t") -> (w4241:string)
                  }
                }
                n3278 = property on="Figure_axis" class="Arr (strict)"("Value"=w4230) -> ()  [unwired: 2 in, 2 out]
                n3279 = property on="data_caption" class="Str"("Value"=w4232) -> ()  [unwired: 2 in, 2 out]
              }
              frame #27 {
                # "2182A 1 channel 2 measure (2182A_1_ch2)"
                n3280 = local read "2182A 1 ch2"() -> (w4249:bool)
                n3281 = property on="Figure_axis" class="Arr (strict)"() -> ("Value"=w4246:string[])  [unwired: 2 in, 2 out]
                n3282 = property on="data_caption" class="Str"() -> ("Value"=w4248:string)  [unwired: 2 in, 2 out]
                n3283 = case shown="True" w4249 {
                  tunnel: w4248 -> [w4251 w4257]
                  tunnel: [w4251 w4256] -> w4247
                  tunnel: w4246 -> [w4250 w4254]
                  tunnel: [w4250 w4252] -> w4245
                  frame False {
                    # "not measure 2182A 1 channel 2 (2182A_1_ch2)"
                  }
                  frame True {
                    w4253 = "2182A_1_ch2"
                    # "measure 2182A 1 channel 2 (2182A_1_ch2)"
                    n3284 = local read "2182A 1 addr"() -> (w4258:u8)
                    n3285 = Number To Decimal String(number=w4258) -> (decimal integer string=w4259:string)  [unwired: 1 in]
                    n3286 = GPIB Clear(3:w4259) -> ()  [unwired: 1 in, 2 out]
                    n3287 = Build Array (concatenate)(w4254, w4253) -> (w4252:string[])
                    n3288 = Concatenate Strings(w4257, w4253, "\t") -> (w4256:string)
                  }
                }
                n3289 = property on="Figure_axis" class="Arr (strict)"("Value"=w4245) -> ()  [unwired: 2 in, 2 out]
                n3290 = property on="data_caption" class="Str"("Value"=w4247) -> ()  [unwired: 2 in, 2 out]
              }
              frame #28 {
                # "2182A 2 channel 1 measure (2182A_2_ch1)"
                n3291 = local read "2182A 2 ch1"() -> (w4264:bool)
                n3292 = property on="Figure_axis" class="Arr (strict)"() -> ("Value"=w4261:string[])  [unwired: 2 in, 2 out]
                n3293 = property on="data_caption" class="Str"() -> ("Value"=w4263:string)  [unwired: 2 in, 2 out]
                n3294 = case shown="True" w4264 {
                  tunnel: w4263 -> [w4266 w4272]
                  tunnel: [w4266 w4271] -> w4262
                  tunnel: w4261 -> [w4265 w4269]
                  tunnel: [w4265 w4267] -> w4260
                  frame False {
                    # "not measure 2182A 2 channel 1 (2182A_2_ch1)"
                  }
                  frame True {
                    w4268 = "2182A_2_ch1"
                    # "measure 2182A 2 channel 1 (2182A_2_ch1)"
                    n3295 = local read "2182A 2 addr"() -> (w4273:u8)
                    n3296 = Number To Decimal String(number=w4273) -> (decimal integer string=w4274:string)  [unwired: 1 in]
                    n3297 = GPIB Clear(3:w4274) -> ()  [unwired: 1 in, 2 out]
                    n3298 = Build Array (concatenate)(w4269, w4268) -> (w4267:string[])
                    n3299 = Concatenate Strings(w4272, w4268, "\t") -> (w4271:string)
                  }
                }
                n3300 = property on="Figure_axis" class="Arr (strict)"("Value"=w4260) -> ()  [unwired: 2 in, 2 out]
                n3301 = property on="data_caption" class="Str"("Value"=w4262) -> ()  [unwired: 2 in, 2 out]
              }
              frame #29 {
                # "2182A 2 channel 2 measure (2182A_2_ch2)"
                n3302 = local read "2182A 2 ch2"() -> (w4279:bool)
                n3303 = property on="Figure_axis" class="Arr (strict)"() -> ("Value"=w4276:string[])  [unwired: 2 in, 2 out]
                n3304 = property on="data_caption" class="Str"() -> ("Value"=w4278:string)  [unwired: 2 in, 2 out]
                n3305 = case shown="True" w4279 {
                  tunnel: w4278 -> [w4281 w4287]
                  tunnel: [w4281 w4286] -> w4277
                  tunnel: w4276 -> [w4280 w4284]
                  tunnel: [w4280 w4282] -> w4275
                  frame False {
                    # "not measure 2182A 2 channel 2 (2182A_2_ch2)"
                  }
                  frame True {
                    w4283 = "2182A_2_ch2"
                    # "measure 2182A 2 channel 2 (2182A_2_ch2)"
                    n3306 = local read "2182A 2 addr"() -> (w4288:u8)
                    n3307 = Number To Decimal String(number=w4288) -> (decimal integer string=w4289:string)  [unwired: 1 in]
                    n3308 = GPIB Clear(3:w4289) -> ()  [unwired: 1 in, 2 out]
                    n3309 = Build Array (concatenate)(w4284, w4283) -> (w4282:string[])
                    n3310 = Concatenate Strings(w4287, w4283, "\t") -> (w4286:string)
                  }
                }
                n3311 = property on="Figure_axis" class="Arr (strict)"("Value"=w4275) -> ()  [unwired: 2 in, 2 out]
                n3312 = property on="data_caption" class="Str"("Value"=w4277) -> ()  [unwired: 2 in, 2 out]
              }
              frame #30 {
                # "2182A 3 channel 1 measure (2182A_3_ch1)"
                n3313 = local read "2182A 3 ch1"() -> (w4294:bool)
                n3314 = property on="Figure_axis" class="Arr (strict)"() -> ("Value"=w4291:string[])  [unwired: 2 in, 2 out]
                n3315 = property on="data_caption" class="Str"() -> ("Value"=w4293:string)  [unwired: 2 in, 2 out]
                n3316 = case shown="True" w4294 {
                  tunnel: w4293 -> [w4296 w4302]
                  tunnel: [w4296 w4301] -> w4292
                  tunnel: w4291 -> [w4295 w4299]
                  tunnel: [w4295 w4297] -> w4290
                  frame False {
                    # "not measure 2182A 3 channel 1 (2182A_3_ch1)"
                  }
                  frame True {
                    w4298 = "2182A_3_ch1"
                    # "measure 2182A 3 channel 1 (2182A_3_ch1)"
                    n3317 = local read "2182A 3 addr"() -> (w4303:u8)
                    n3318 = Number To Decimal String(number=w4303) -> (decimal integer string=w4304:string)  [unwired: 1 in]
                    n3319 = GPIB Clear(3:w4304) -> ()  [unwired: 1 in, 2 out]
                    n3320 = Build Array (concatenate)(w4299, w4298) -> (w4297:string[])
                    n3321 = Concatenate Strings(w4302, w4298, "\t") -> (w4301:string)
                  }
                }
                n3322 = property on="Figure_axis" class="Arr (strict)"("Value"=w4290) -> ()  [unwired: 2 in, 2 out]
                n3323 = property on="data_caption" class="Str"("Value"=w4292) -> ()  [unwired: 2 in, 2 out]
              }
              frame #31 {
                # "2182A 3 channel 2 measure (2182A_3_ch2)"
                n3324 = local read "2182A 3 ch2"() -> (w4309:bool)
                n3325 = property on="Figure_axis" class="Arr (strict)"() -> ("Value"=w4306:string[])  [unwired: 2 in, 2 out]
                n3326 = property on="data_caption" class="Str"() -> ("Value"=w4308:string)  [unwired: 2 in, 2 out]
                n3327 = case shown="False" w4309 {
                  tunnel: w4308 -> [w4311 w4317]
                  tunnel: [w4311 w4316] -> w4307
                  tunnel: w4306 -> [w4310 w4314]
                  tunnel: [w4310 w4312] -> w4305
                  frame False {
                    # "not measure 2182A 3 channel 2 (2182A_3_ch2)"
                  }
                  frame True {
                    w4313 = "2182A_3_ch2"
                    # "measure 2182A 3 channel 2 (2182A_3_ch2)"
                    n3328 = local read "2182A 3 addr"() -> (w4318:u8)
                    n3329 = Number To Decimal String(number=w4318) -> (decimal integer string=w4319:string)  [unwired: 1 in]
                    n3330 = GPIB Clear(3:w4319) -> ()  [unwired: 1 in, 2 out]
                    n3331 = Build Array (concatenate)(w4314, w4313) -> (w4312:string[])
                    n3332 = Concatenate Strings(w4317, w4313, "\t") -> (w4316:string)
                  }
                }
